vi "sendRunScriptEvent.vi"(8 "error in (no error)":errorcluster, 10 "runSingleScript":cluster{"Path":path, "HWLoop":bool}, 11 "ExperimentControl in":refnum<class "ExperimentControl.lvclass">) -> (0 "error out":errorcluster, 2 "configured":bool, 3 "ExperimentControl out":refnum<class "ExperimentControl.lvclass">)   [LabVIEW 2011, in "Views.lvlib" / "ExperimentControl.lvlib" / "ExperimentControl.lvclass"]
uses:
  ExperimentControl.lvclass
  ExperimentControl.lvclass/ExperimentControl.ctl
  Hal/HWController/HWControllerEvents/HWControllerEvents.lvclass
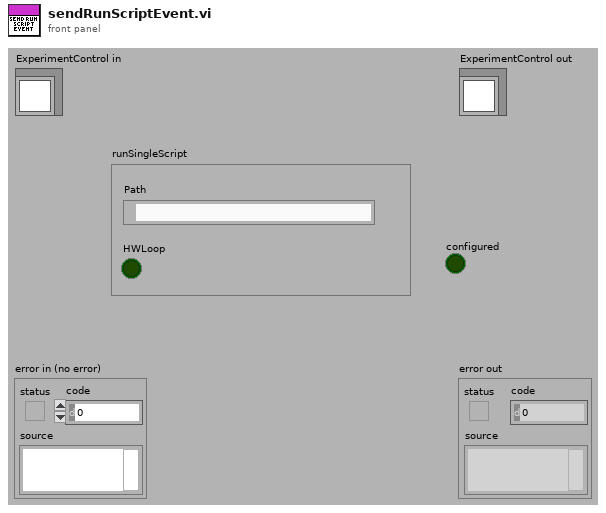
[diagram p1: front panel]
types:
  T1 = enum16{"start", "stop", "statusInquiry", "configure", "resetError", "resourcesInquiry", "reserveResources", "initialise", "resetAllChannels", "staticUpdate", "close", "HWStatus", "error", "resourcesAvailable", "resourcesReserved", "compilerError", "compiledScript", "compilingScript", "runScript", "configureCompiledScript"}
  T2 = enum16{"Ready", "Compiling", "Configured", "Running", "Stopping", "Unresolved Error"}
  T3 = cluster{"incomingEventTypes":cluster{"start":cluster{"Boolean":bool}, "stop":cluster{"Boolean":bool}, "statusInquiry":cluster{"Boolean":bool}, "configure":cluster{"DPScriptPath":path, "TimeStamp":string, "HWLoop?":bool}, "resetError":cluster{"Boolean":bool}, "resourcesInquiry":cluster{"Boolean":bool}, "reserveResources":cluster{"HWList":string[]}, "initialise":cluster{"HWList":string[]}, "close":cluster{"Boolean":bool}, "resetAllChannels":cluster{"Boolean":bool}, "staticChannelUpdate":cluster{"channel_address":string, "calibratedValue":dbl}, "runScript":cluster{"DPScriptPath":path, "TimeStamp":string, "HWLoop?":bool}, "compilingScript":cluster{"Path":path}, "compiledScript":cluster{"Path":path, "timeCompileAt":string}, "compilerError":cluster{"Path":path}, "configureCompiledScript":cluster{"DPScriptPath":path, "TimeStamp":string, "HWLoop?":bool, "CompiledScript":cluster{"ScriptListCompiler.lvclass":refnum<class "ScriptListCompiler.lvclass">, "aoChannels":refnum<class "AnalogOutput.lvclass">[], "doChannels":refnum<class "DigitalOutput.lvclass">[], "rfChannels":refnum<class "DDSOutput.lvclass">[]}}, "restartCompiler":cluster{"restart":bool}, "staticRfChannelUpdate":cluster{"channel_address":string, "Output":cluster{"Frequency(MHz)":dbl, "Amplitude":dbl, "Phase":dbl, "OutputForm":enum16{"Sine", "Square", "Triangle", "Arbitrary"}}}, "cameraUpdate":cluster{"Camera":string, "Type":string, "settings":path}}, "outgoingEventTypes":cluster{"HWStatus":cluster{"status":enum16{"Ready", "Compiling", "Configured", "Running", "Stopping", "Unresolved Error"}}, "error":cluster{"error out":errorcluster}, "resourcesAvailable":cluster{"availableHWList":string[], "reservedHWList":string[]}, "resourcesReserved":cluster{"reservedHWList":string[]}}}
  T4 = cluster{"status":enum16{"Ready", "Compiling", "Configured", "Running", "Stopping", "Unresolved Error"}}
  T5 = cluster{"DPScriptPath":path, "TimeStamp":string, "HWLoop?":bool}
  T6 = enum16{"start", "stop", "statusInquiry", "configure", "resetError", "resourcesInquiry", "reserveResources", "initialise", "resetAllChannels", "staticUpdate", "close", "HWStatus", "error", "resourcesAvailable", "resourcesReserved", "compilerError", "compiledScript", "compilingScript", "runScript", "configureCompiledScript", "restartCompiler", "staticRfChannelUpdate", "cameraUpdate"}
  T7 = cluster{"eventId":enum16{"start", "stop", "statusInquiry", "configure", "resetError", "resourcesInquiry", "reserveResources", "initialise", "resetAllChannels", "staticUpdate", "close", "HWStatus", "error", "resourcesAvailable", "resourcesReserved", "compilerError", "compiledScript", "compilingScript", "runScript", "configureCompiledScript"}, "runScript":cluster{"DPScriptPath":path, "TimeStamp":string, "HWLoop?":bool}}
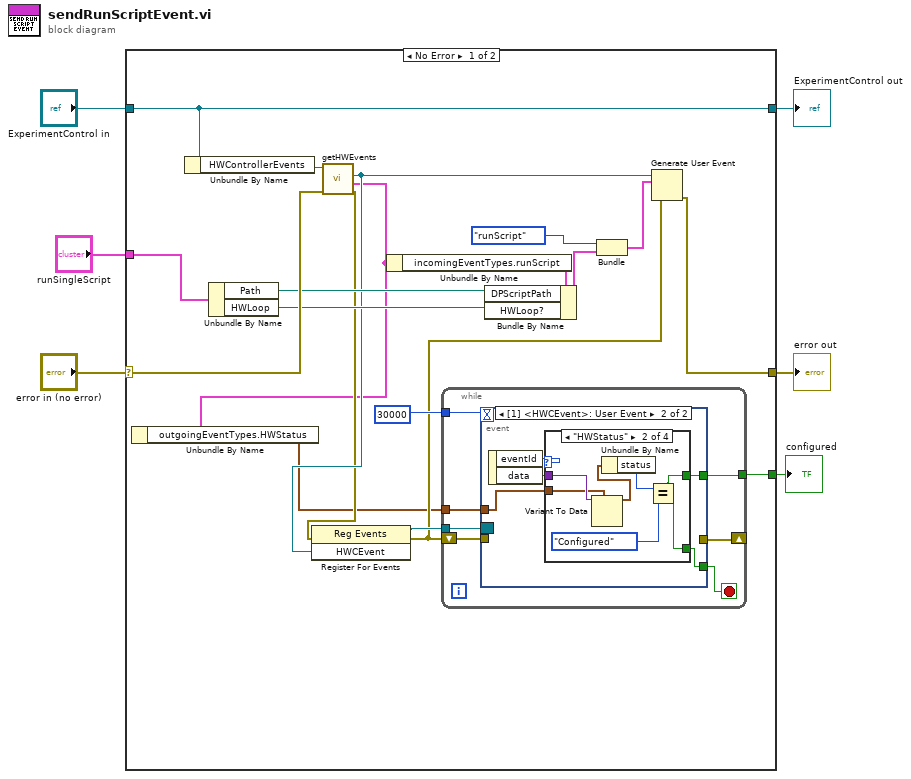
[diagram p0: block diagram]
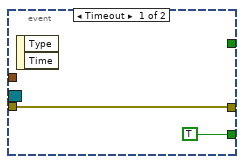
[diagram p2: hidden frame]
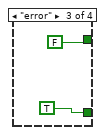
[diagram p4: hidden frame]
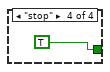
[diagram p5: hidden frame]
diagram:
  n1 = case shown="No Error" "error in (no error)" {
    selector: "error in (no error)" -> [w23 w50]
    tunnel: [w18 w50] -> w5
    tunnel: [w25 w49] -> w3
    tunnel: "ExperimentControl in" -> [w25 w49]
    tunnel: "runSingleScript" -> [w17 _]
    tunnel: [w9 _] -> w1
    frame No Error {
      n2 = Unbundle By Name(w25) -> ("HWControllerEvents"=w24:refnum<class "HWControllerEvents.lvclass">)
      n3 = Unbundle By Name(w17) -> ("Path"=w16:path, "HWLoop"=w15:bool)
      n4 = call-dynamic "getHWEvents.vi"("error in (no error)"=w23, "HWControllerEvents in"=w24) -> ("error out"=w11:errorcluster, "eventDataTypes"=w7:T3, "HWCEvent"=w14:refnum<user-event>)  [unwired: 6 in, 1 out]
      n5 = Unbundle By Name(w7) -> ("outgoingEventTypes.HWStatus"=w8:T4)
      n6 = register-events(error in=w11, w14) -> (reference out=w13:refnum<event-registration>, error out=w10:errorcluster)  [unwired: 1 in]
      n7 = Unbundle By Name(w7) -> ("incomingEventTypes.runScript"=w22:T5)
      n8 = while {
        tunnel: w13 -> [w32]
        shift-right: [w28] -> _
        shift-left: w10 -> [w31]
        tunnel: 30000 -> [w30]
        tunnel: [w27] -> w9
        tunnel: w8 -> [w26]
        stop <- w29 stop-if-true
        n9 = event shown="[1] <HWCEvent>: User Event" {
          selector: w32 -> [_ _]
          dyn-events: _ -> [_ _]
          timeout: w30 -> [_ _]
          tunnel: w31 -> [w33 _]
          tunnel: [TRUE w38] -> w29
          tunnel: [w33 _] -> w28
          tunnel: [_ w37] -> w27
          tunnel: w26 -> [_ w35]
          event Timeout {
            n10 = event-data() -> ()  [unwired: 1 in, 2 out]
          }
          event User Event {
            n11 = event-data() -> ("eventId"=w39:T6, "data"=w36:variant)  [unwired: 1 in]
            n12 = case shown="\"HWStatus\"" w39 {
              tunnel: [_ w40 TRUE TRUE] -> w38
              tunnel: [_ w40 FALSE _] -> w37
              tunnel: w36 -> [_ w45 _ _]
              tunnel: w35 -> [_ w44 _ _]
              frame Default {
              }
              frame "HWStatus" {
                n13 = Variant To Data(type=w44, Variant=w45) -> (data=w43:T4)  [unwired: 1 in, 1 out]
                n14 = Unbundle By Name(w43) -> ("status"=w42:T2)
                n15 = Equal?(x=w42, y=T2."Configured") -> (x = y?=w40:bool)
              }
              frame "error" {
              }
              frame "stop" {
              }
            }
          }
        }
      }
      n16 = Bundle By Name(cluster=w22, "DPScriptPath"=w16, "HWLoop?"=w15) -> (w21:T5)
      n17 = Bundle("eventId"=T1."runScript", "runScript"=w21) -> (w19:T7)  [unwired: 1 in]
      n18 = Generate User Event(user event=w14, event data cluster=w19, error in=w10) -> (error out=w18:errorcluster)  [unwired: 1 out]
    }
    frame Error {
    }
  }
  "error out" <- w5
  "ExperimentControl out" <- w3
  "configured" <- w1
